vi "RCV Test_Hold and Measure Over Time_ksENA.vi"(0 "Semiconductor Module Context":T3, 1 "Hold Time(s)":dbl=1.0, 2 "Test Information":T6={"Exp Name"="Cold Switching", "Lot"="0233A", "Wafer"="15", "Die Type"="L22", "Die X "="6", "Die Y"="8", "Exp"="1", "Die X_Y"="8"}, 3 "# of Cycles":string, 5 "Sweep Settings":T4={"Start"=0.0, "Stop"=1.0, "Step"=0.0}, 7 "Test_Pins":T5={"RF_Pins"=["RF1", "RF2"], "Contact_Meas_Pins"=["RF1"], "Contact_Source_Pins"=["RF1"], "Sweep_Bias_Pins"=[]}, 9 "Averaging Count":i32=3, 11 "error in (no error)":errorcluster, 12 "Meas Type":T1, 13 "base path":path=path "C:/Users/Eddie.Rickey/Desktop/Test Data/Plots", 14 "Hold Down Current level":dbl=0.001 format="%#_13p") -> (4 "Time":dbl[](array[numeric]), 6 "ks5080A_Meaurements":T7, 15 "error out":errorcluster)   [LabVIEW 2013]
doc: "Initiates and fetches niVNA S11 measurements and converts it to a capacitance measurement."
uses:
  <vilib>/NI_TestStand_SemiconductorModule/NI_TestStand_Semiconductor_Module.lvlibp/PinMap/General/SemiconductorModuleContext.ctl
  Controls/Sweep Settings.ctl
  Controls/Test_Pins.ctl
  Controls/Test Information.ctl
  Controls/Meas Type.ctl
  Controls/ks5080A_Measurements.ctl
  <vilib>/NI_TestStand_SemiconductorModule/NI_TestStand_Semiconductor_Module.lvlibp
panel:
  in  "Tab Control":enum32{"Graphs", "Inputs", "Outputs"}(tab)
  out "Resistance over time":cluster{dbl[], dbl[]}(graph)
  out "Port Capacitance over time":cluster{dbl[], "P2_Capacitance":dbl[]}[](graph)
  out "Graph Cluster":T2
  out "Die Type":string
  out "Measurement":string
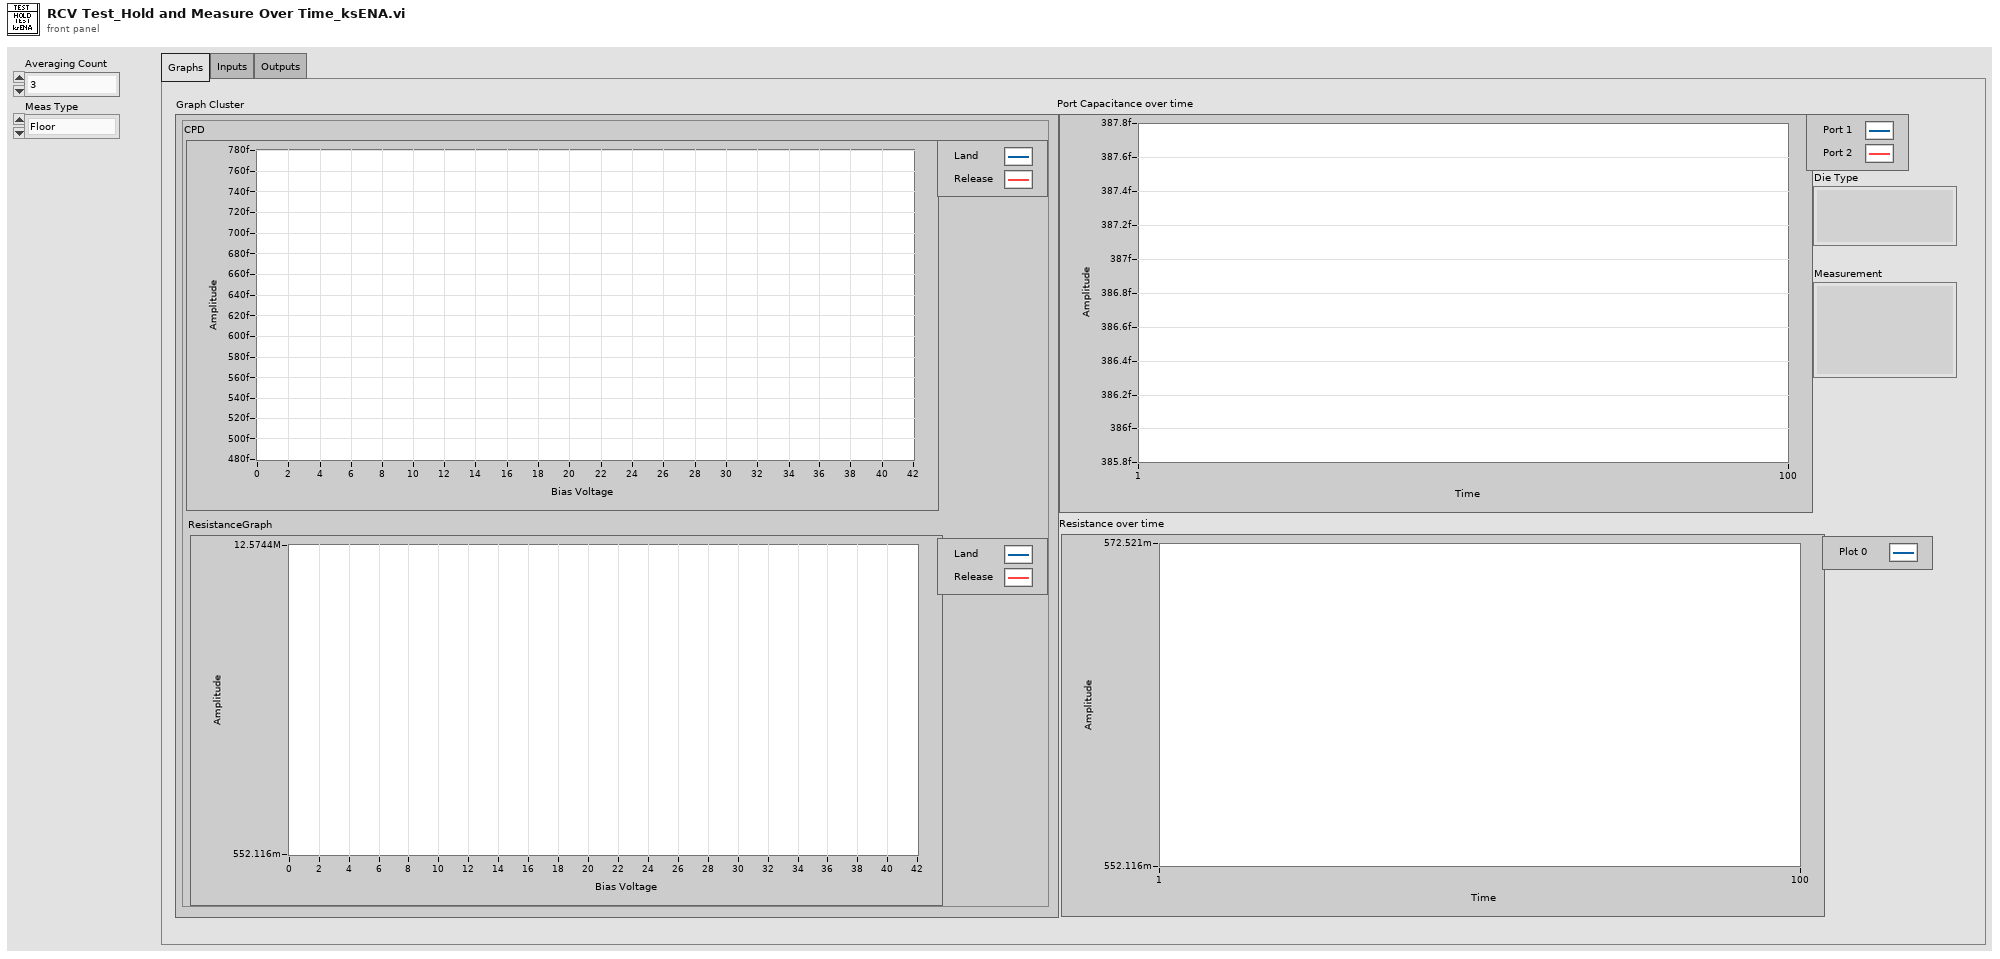
[diagram p1: front panel]
types:
  T1 = typedef "Meas Type.ctl" = enum16{"Floor", "Roof", "Buckling", "Charge Transfer"}
  T2 = cluster{"ResistanceGraph":cluster{dbl[], dbl[]}[], "CPD":cluster{dbl[], dbl[]}[]}
  T3 = typedef "NI_TestStand_Semiconductor_Module.lvlibp/SemiconductorModuleContext.ctl" = refnum<k7>
  T4 = typedef "Sweep Settings.ctl" = cluster{"Start":dbl, "Stop":dbl, "Step":dbl}
  T5 = typedef "Test_Pins.ctl" = cluster{"RF_Pins":string[], "Contact_Meas_Pins":string[], "Contact_Source_Pins":string[], "Sweep_Bias_Pins":string[]}
  T6 = typedef "Test Information.ctl" = cluster{"Exp Name":string, "Lot":string, "Wafer":string, "Die Type":string, "Die X ":string, "Die Y":string, "Exp":string, "Die X_Y":string}
  T7 = typedef "ks5080A_Measurements.ctl" = cluster{"Bias_Sweep_Setting":dbl[], "Bias_voltage measurements":dbl[], "Bias_current measurements":dbl[], "P1_Capacitance":dbl[], "P2_Capacitance":dbl[], "DMM_Measurement_V":dbl[], "Contact_Source Current measurements":dbl[], "Contact_Sink Current measurements":dbl[], "Calculated_Resistance":dbl[], "P3_Capacitance":dbl[], "Port 1_S_parm":string[], "Port 2_S_parm":string[], "Port 3_S_parm":string[]}
  T8 = enum16{"Initialize", "Insert Data into Array", "Get Data"}
  T9 = typedef "ENA_Marker Measurements.ctl" = cluster{"Port 1 Capacitance":dbl[], "Port 2 Capacitance":dbl[], "Port 3 Capacitance":dbl[], "Port 1_S_parm":string[], "Port 2_S_parm":string[], "Port 3_S_parm":string[]}
  T10 = typedef "imagedata.ctl" = cluster{"image type":i32, "image depth":i32, "image":u8[], "mask":u8[], "colors":u32[], "Rectangle":cluster{"left":i16, "top":i16, "right":i16, "bottom":i16}}
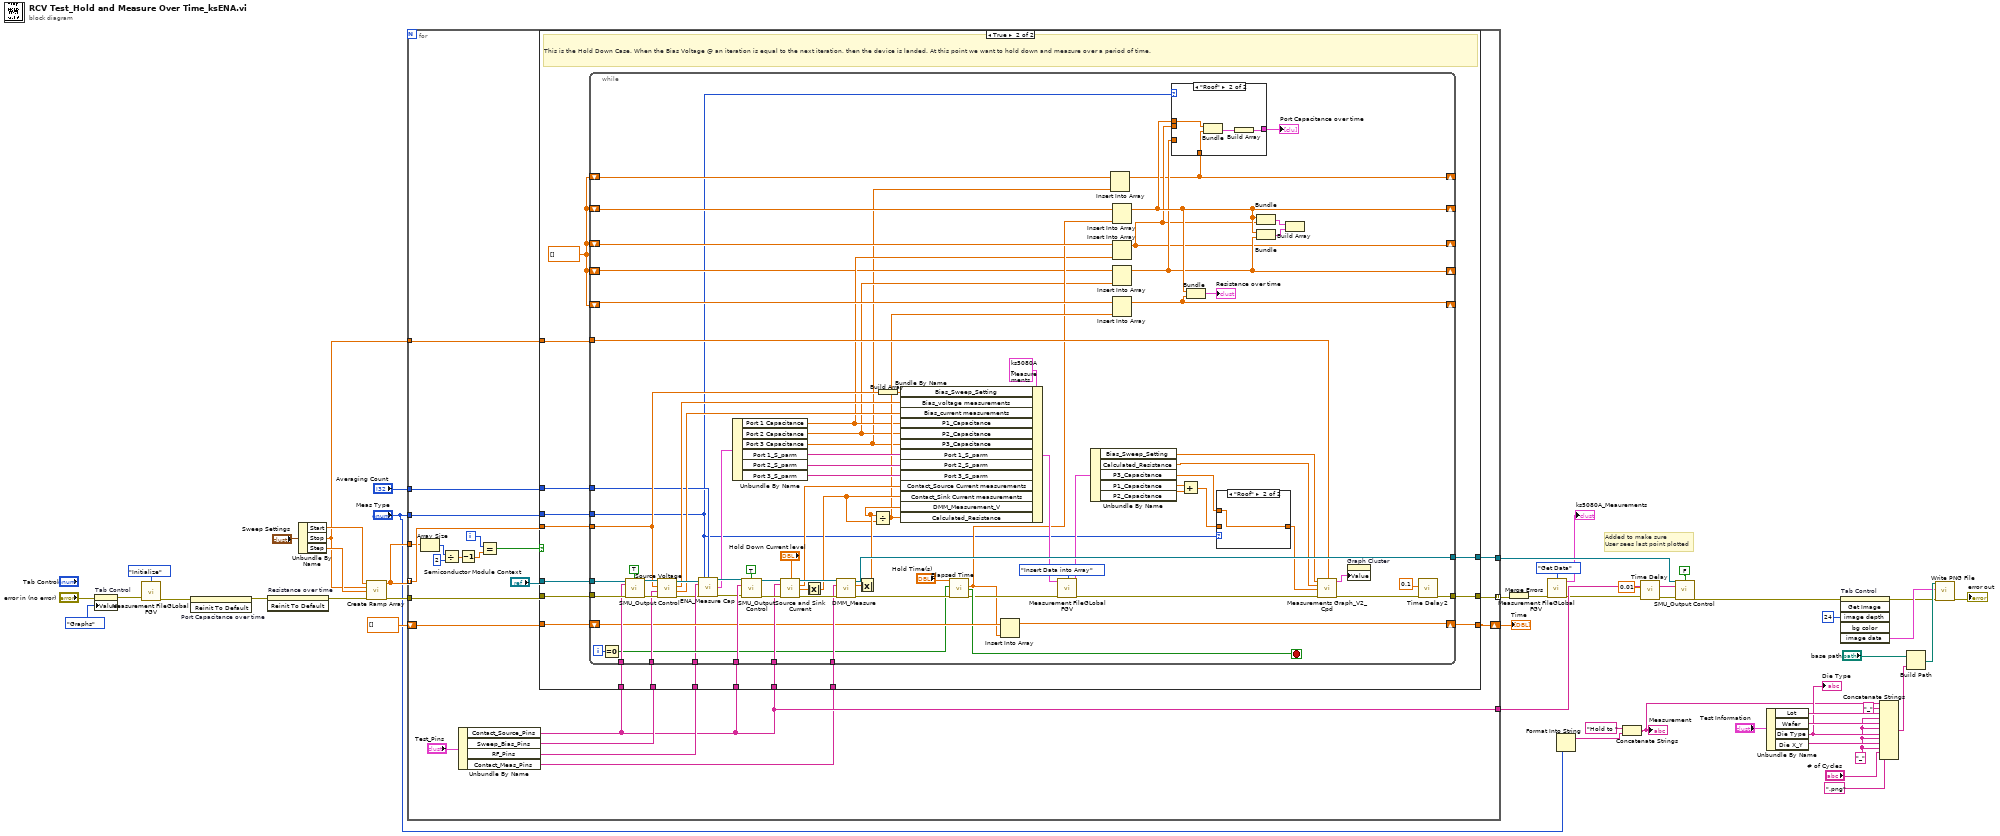
[diagram p0: block diagram]
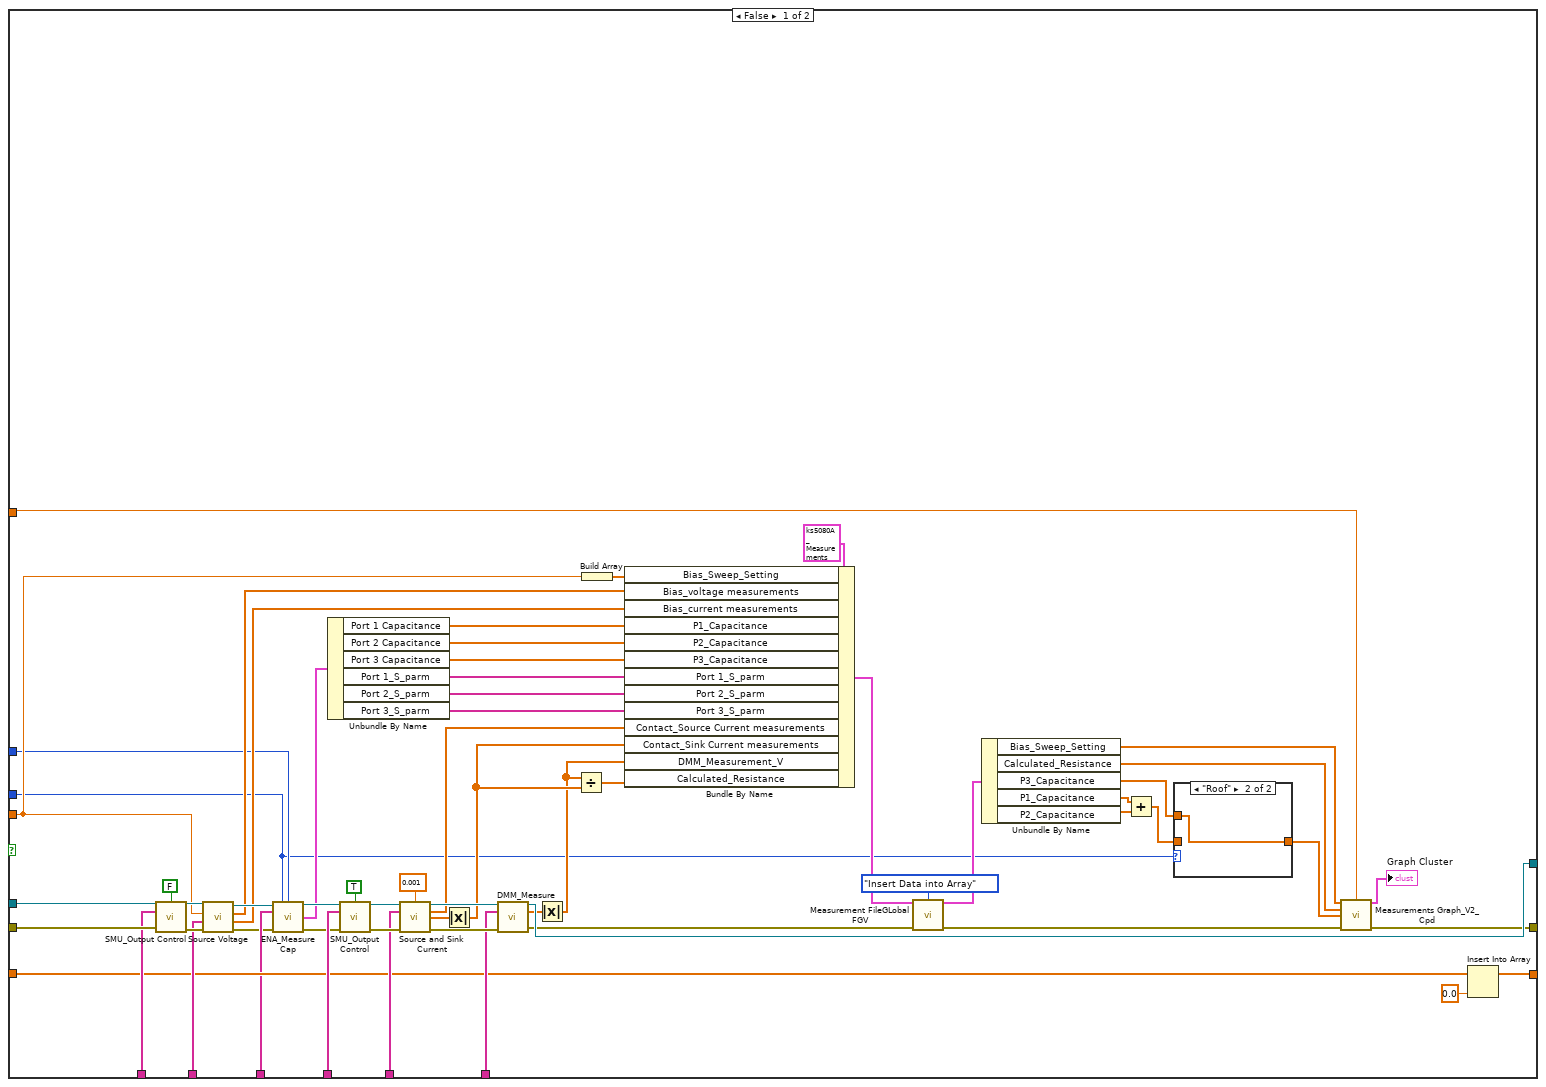
[diagram p2: hidden frame]
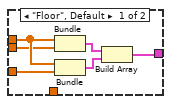
[diagram p4: hidden frame]
diagram:
  w3 = "_"
  # "Added to make sure \nUser sees last point plotted"
  n1 = property on="Tab Control" class="TabCtl (strict)"(error in="error in (no error)", "Value"=enum32{"Graphs", "Inputs", "Outputs"}."Graphs" ("Tab Control")) -> (error out=w14:errorcluster)  [unwired: 1 in, 1 out]
  n2 = call "Measurement FileGLobal FGV.vi"("Enum"=T8."Initialize", "Error In"=w14) -> ("Error Out"=w24:errorcluster)  [unwired: 12 in, 1 out]
  n3 = invoke on="Port Capacitance over time" class="XYGraph (strict)" method="Reinit To Default"(error in=w24) -> (error out=w26:errorcluster)  [unwired: 2 in, 2 out]
  n4 = invoke on="Resistance over time" class="XYGraph (strict)" method="Reinit To Default"(error in=w26) -> (error out=w25:errorcluster)  [unwired: 2 in, 2 out]
  n5 = Unbundle By Name("Sweep Settings") -> ("Start"=w45:dbl, "Stop"=w31:dbl, "Step"=w44:dbl)
  n6 = call "Create Ramp Array.vi"("Start"=w45, "Stop"=w31, "Step"=w44, "Error In"=w25) -> ("Ramp Pattern"=w27:dbl[], "Error Out"=w47:errorcluster)  [unwired: 10 in]
  n7 = for {
    tunnel: w27 -> [w58] mode=indexing
    tunnel: [w67] -> w20 mode=indexing
    tunnel: w47 -> [w68]
    tunnel: w31 -> [w57]
    tunnel: [w63] -> w30
    tunnel: [w61] -> w29
    shift-right: [w60] -> w28
    shift-left: dbl[] [] -> [w59]
    tunnel: w27 -> [w56]
    tunnel: "Averaging Count" -> [w49]
    tunnel: "Meas Type" -> [w48]
    i -> [w51]
    n8 = Array Size(array=w56) -> (size(s)=w55:i32)
    n9 = Divide(x=w55, y=2) -> (x/y=w53:dbl)
    n10 = Unbundle By Name("Test_Pins") -> ("Contact_Source_Pins"=w63:string[], "Sweep_Bias_Pins"=w65:string[], "RF_Pins"=w64:string[], "Contact_Meas_Pins"=w62:string[])
    n11 = Decrement(x=w53) -> (x-1=w52:dbl)
    n12 = Equal?(x=w51, y=w52) -> (x = y?=w50:bool)
    n13 = case shown="True" w50 {
      tunnel: [w82 w147] -> w67
      tunnel: w68 -> [w120 w148]
      tunnel: w58 -> [w100 w146]
      tunnel: w57 -> [w81 w145]
      tunnel: "Semiconductor Module Context" -> [w119 w144]
      tunnel: w63 -> [w117 w143]
      tunnel: w65 -> [w116 w142]
      tunnel: w64 -> [w107 w141]
      tunnel: w63 -> [w115 w140]
      tunnel: w63 -> [w114 w139]
      tunnel: w62 -> [w113 w138]
      tunnel: [w118 w137] -> w61
      tunnel: [w112 w136] -> w60
      tunnel: w59 -> [w111 w135]
      tunnel: w49 -> [w72 w134]
      tunnel: w48 -> [w71 w133]
      frame False {
        n14 = call "SMU_Output Control.vi"("Semiconductor Module Context"=w119, "output enabled?"=FALSE, "Pins"=w117, "error in (no error)"=w120) -> ("Semiconductor Module Context Out"=w128:T3, "error out"=w129:errorcluster)  [unwired: 10 in]
        n15 = call "Source Voltage.vi"("error in (no error)"=w129, "Pins"=w116, "voltage level"=w100, "Semiconductor Module Context"=w128) -> ("error out"=w106:errorcluster, "current measurements"=w97:dbl[], "voltage measurements"=w98:dbl[], "Semiconductor Module Context Out"=w103:T3)  [unwired: 4 in]
        n16 = call "ENA_Measure Cap.vi"("Semiconductor Module Context"=w103, "Meas Type"=w71, "Averaging Count"=w72, "Pins"=w107, "error in (no error)"=w106) -> ("Semiconductor Module Context Out"=w104:T3, "Marker Measurements"=w102:T9, "error out"=w105:errorcluster)  [unwired: 8 in]
        n17 = Unbundle By Name(w102) -> ("Port 1 Capacitance"=w95:dbl[], "Port 2 Capacitance"=w94:dbl[], "Port 3 Capacitance"=w93:dbl[], "Port 1_S_parm"=w92:string[], "Port 2_S_parm"=w91:string[], "Port 3_S_parm"=w90:string[])
        n18 = call "SMU_Output Control.vi"("Semiconductor Module Context"=w104, "output enabled?"=TRUE, "Pins"=w115, "error in (no error)"=w105) -> ("Semiconductor Module Context Out"=w121:T3, "error out"=w122:errorcluster)  [unwired: 10 in]
        n19 = call "Source and Sink Current.vi"("Semiconductor Module Context"=w121, "Current level"=0.001, "Pins"=w114, "error in (no error)"=w122) -> ("Semiconductor Module Context Out"=w123:T3, "Source Current measurements"=w89:dbl[], "Sink Current measurements"=w109:dbl[], "error out"=w124:errorcluster)  [unwired: 8 in]
        n20 = Absolute Value(x=w109) -> (abs(x)=w88:dbl[])
        n21 = call "DMM_Measure.vi"("Semiconductor Module Context"=w123, "Pins"=w113, "Error In"=w124) -> ("Semiconductor Module Context Out"=w118:T3, "Measurement"=w108:dbl[], "Error Out"=w86:errorcluster)  [unwired: 10 in]
        n22 = Absolute Value(x=w108) -> (abs(x)=w84:dbl[])
        n23 = Divide(x=w84, y=w88) -> (x/y=w87:dbl[])
        n24 = Build Array(w100) -> (w99:dbl[])
        n25 = Bundle By Name(cluster=T7 {"Bias_Sweep_Setting"=[], "Bias_voltage measurements"=[], "Bias_current measurements"=[], "P1_Capacitance"=[], "P2_Capacitance"=[], "DMM_Measurement_V"=[], "Contact_Source Current measurements"=[], "Contact_Sink Current measurements"=[], "Calculated_Resistance"=[], "P3_Capacitance"=[], "Port 1_S_parm"=[], "Port 2_S_parm"=[], "Port 3_S_parm"=[]} ("ks5080A_Meaurements"), "Bias_Sweep_Setting"=w99, "Bias_voltage measurements"=w98, "Bias_current measurements"=w97, "P1_Capacitance"=w95, "P2_Capacitance"=w94, "P3_Capacitance"=w93, "Port 1_S_parm"=w92, "Port 2_S_parm"=w91, "Port 3_S_parm"=w90, "Contact_Source Current measurements"=w89, "Contact_Sink Current measurements"=w88, "DMM_Measurement_V"=w84, "Calculated_Resistance"=w87) -> (w96:T7)
        n26 = call "Measurement FileGLobal FGV.vi"("New Measurements"=w96, "Enum"=T8."Insert Data into Array", "Error In"=w86) -> ("Combined Measurements"=w85:T7, "Error Out"=w83:errorcluster)  [unwired: 11 in]
        n27 = Unbundle By Name(w85) -> ("Bias_Sweep_Setting"=w79:dbl[], "Calculated_Resistance"=w78:dbl[], "P3_Capacitance"=w73:dbl[], "P1_Capacitance"=w77:dbl[], "P2_Capacitance"=w76:dbl[])
        n28 = Add(x=w77, y=w76) -> (x+y=w75:dbl[])
        n29 = case shown="\"Roof\"" w71 {
          tunnel: w75 -> [w130 _]
          tunnel: [w130 w131] -> w74
          tunnel: w73 -> [_ w131]
          frame "Floor", Default {
          }
          frame "Roof" {
          }
        }
        n30 = call "Measurements Graph_V2_Cpd.vi"("Bias Voltage"=w79, "Stop_V"=w81, "Resitance"=w78, "Cpd"=w74, "Error In"=w83) -> ("Graph Cluster"=→"Graph Cluster":T2, "Error Out"=w82:errorcluster)  [unwired: 9 in]
        n31 = Insert Into Array(array=w111, new element=0.0 ("new element/subarray")) -> (w112:dbl[])  [unwired: 1 in]
      }
      frame True {
        w132 = dbl[] []
        # "This is the Hold Down Case. When the Bias Voltage @ an iteration is equal to the next iteration, then the device is landed. At this point we want to hold down and measure over a period of time."
        n32 = while {
          tunnel: [w210] -> w147
          tunnel: w148 -> [w219]
          tunnel: w146 -> [w190]
          tunnel: w145 -> [w174]
          tunnel: w144 -> [w218]
          tunnel: w143 -> [w217]
          tunnel: w142 -> [w216]
          tunnel: w141 -> [w197]
          tunnel: w140 -> [w215]
          tunnel: w139 -> [w214]
          tunnel: w138 -> [w213]
          tunnel: [w212] -> w137
          shift-right: [w200] -> w136
          shift-left: w135 -> [w209]
          shift-right: [w161] -> _
          shift-left: w132 -> [w202]
          shift-right: [w155] -> _
          shift-left: w132 -> [w201]
          shift-right: [w157] -> _
          shift-left: w132 -> [w165]
          tunnel: w134 -> [w159]
          tunnel: w133 -> [w151]
          shift-right: [w156] -> _
          shift-left: w132 -> [w163]
          shift-right: [w152] -> _
          shift-left: w132 -> [w154]
          i -> [w206]
          stop <- w208 stop-if-true
          n33 = Equal To 0?(x=w206) -> (x = 0?=w205:bool)
          n34 = call "SMU_Output Control.vi"("Semiconductor Module Context"=w218, "output enabled?"=TRUE, "Pins"=w217, "error in (no error)"=w219) -> ("Semiconductor Module Context Out"=w228:T3, "error out"=w229:errorcluster)  [unwired: 10 in]
          n35 = call "Source Voltage.vi"("error in (no error)"=w229, "Pins"=w216, "voltage level"=w190, "Semiconductor Module Context"=w228) -> ("error out"=w149:errorcluster, "current measurements"=w192:dbl[], "voltage measurements"=w193:dbl[], "Semiconductor Module Context Out"=w195:T3)  [unwired: 4 in]
          n36 = call "ENA_Measure Cap.vi"("Semiconductor Module Context"=w195, "Meas Type"=w151, "Averaging Count"=w159, "Pins"=w197, "error in (no error)"=w149) -> ("Semiconductor Module Context Out"=w194:T3, "Marker Measurements"=w189:T9, "error out"=w196:errorcluster)  [unwired: 8 in]
          n37 = Unbundle By Name(w189) -> ("Port 1 Capacitance"=w164:dbl[], "Port 2 Capacitance"=w162:dbl[], "Port 3 Capacitance"=w153:dbl[], "Port 1_S_parm"=w188:string[], "Port 2_S_parm"=w187:string[], "Port 3_S_parm"=w186:string[])
          n38 = call "SMU_Output Control.vi"("Semiconductor Module Context"=w194, "output enabled?"=TRUE, "Pins"=w215, "error in (no error)"=w196) -> ("Semiconductor Module Context Out"=w221:T3, "error out"=w222:errorcluster)  [unwired: 10 in]
          n39 = call "Source and Sink Current.vi"("Semiconductor Module Context"=w221, "Current level"="Hold Down Current level", "Pins"=w214, "error in (no error)"=w222) -> ("Semiconductor Module Context Out"=w223:T3, "Source Current measurements"=w185:dbl[], "Sink Current measurements"=w204:dbl[], "error out"=w224:errorcluster)  [unwired: 8 in]
          n40 = Absolute Value(x=w204) -> (abs(x)=w183:dbl[])
          n41 = call "DMM_Measure.vi"("Semiconductor Module Context"=w223, "Pins"=w213, "Error In"=w224) -> ("Semiconductor Module Context Out"=w212:T3, "Measurement"=w203:dbl[], "Error Out"=w220:errorcluster)  [unwired: 10 in]
          n42 = Absolute Value(x=w203) -> (abs(x)=w184:dbl[])
          n43 = Divide(x=w184, y=w183) -> (x/y=w169:dbl[])
          n44 = Build Array(w190) -> (w191:dbl[])
          n45 = Bundle By Name(cluster=T7 {"Bias_Sweep_Setting"=[], "Bias_voltage measurements"=[], "Bias_current measurements"=[], "P1_Capacitance"=[], "P2_Capacitance"=[], "DMM_Measurement_V"=[], "Contact_Source Current measurements"=[], "Contact_Sink Current measurements"=[], "Calculated_Resistance"=[], "P3_Capacitance"=[], "Port 1_S_parm"=[], "Port 2_S_parm"=[], "Port 3_S_parm"=[]} ("ks5080A_Meaurements"), "Bias_Sweep_Setting"=w191, "Bias_voltage measurements"=w193, "Bias_current measurements"=w192, "P1_Capacitance"=w164, "P2_Capacitance"=w162, "P3_Capacitance"=w153, "Port 1_S_parm"=w188, "Port 2_S_parm"=w187, "Port 3_S_parm"=w186, "Contact_Source Current measurements"=w185, "Contact_Sink Current measurements"=w183, "DMM_Measurement_V"=w184, "Calculated_Resistance"=w169) -> (w182:T7)
          n46 = call "Elapsed Time"("Time Target (s)"="Hold Time(s)", "Reset"=w205, "error in (no error)"=w220) -> ("Elapsed Time (s)"=w167:dbl, "Time has Elapsed"=w208:bool, "error out"=w199:errorcluster)  [unwired: 9 in, 5 out]
          n47 = Insert Into Array(array=w209, new element=w167) -> (w200:dbl[])  [unwired: 1 in]
          n48 = call "Measurement FileGLobal FGV.vi"("New Measurements"=w182, "Enum"=T8."Insert Data into Array", "Error In"=w199) -> ("Combined Measurements"=w173:T7, "Error Out"=w177:errorcluster)  [unwired: 11 in]
          n49 = Unbundle By Name(w173) -> ("Bias_Sweep_Setting"=w172:dbl[], "Calculated_Resistance"=w171:dbl[], "P3_Capacitance"=w178:dbl[], "P1_Capacitance"=w181:dbl[], "P2_Capacitance"=w180:dbl[])
          n50 = Insert Into Array(array=w154, new element=w153) -> (w152:dbl[])  [unwired: 1 in]
          n51 = Insert Into Array(array=w165, new element=w167) -> (w157:dbl[])  [unwired: 1 in]
          n52 = Insert Into Array(array=w201, new element=w164) -> (w155:dbl[])  [unwired: 1 in]
          n53 = Insert Into Array(array=w163, new element=w162) -> (w156:dbl[])  [unwired: 1 in]
          n54 = Insert Into Array(array=w202, new element=w169) -> (w161:dbl[])  [unwired: 1 in]
          n55 = case shown="\"Roof\"" w151 {
            tunnel: [w233 w238] -> w158
            tunnel: w157 -> [w232 w237]
            tunnel: w155 -> [w231 _]
            tunnel: w156 -> [w230 _]
            tunnel: w152 -> [_ w236]
            frame "Floor", Default {
              n56 = Bundle(w232, w231) -> (w235:cluster{dbl[], dbl[]})  [unwired: 1 in]
              n57 = Bundle(w232, w230) -> (w234:cluster{dbl[], dbl[]})  [unwired: 1 in]
              n58 = Build Array(w235, w234) -> (w233:cluster{dbl[], dbl[]}[])
            }
            frame "Roof" {
              n59 = Bundle(w237, w236) -> (w239:cluster{dbl[], dbl[]})  [unwired: 1 in]
              n60 = Build Array(w239) -> (w238:cluster{dbl[], dbl[]}[])
            }
          }
          "Port Capacitance over time" <- w158
          n61 = Add(x=w181, y=w180) -> (x+y=w179:dbl[])
          n62 = Bundle(w157, w161) -> (→"Resistance over time":cluster{dbl[], dbl[]})  [unwired: 1 in]
          n63 = case shown="\"Roof\"" w151 {
            tunnel: w179 -> [w240 _]
            tunnel: [w240 w241] -> w170
            tunnel: w178 -> [_ w241]
            frame "Floor", Default {
            }
            frame "Roof" {
            }
          }
          n64 = Bundle(w157, w155) -> (w168:cluster{dbl[], dbl[]})  [unwired: 1 in]
          n65 = Bundle(w157, w156) -> (w166:cluster{dbl[], dbl[]})  [unwired: 1 in]
          n66 = Build Array(w168, w166) -> ()  [unwired: 1 out]
          n67 = call "Measurements Graph_V2_Cpd.vi"("Bias Voltage"=w172, "Stop_V"=w174, "Resitance"=w171, "Cpd"=w170, "Error In"=w177) -> ("Graph Cluster"=w175:T2, "Error Out"=w176:errorcluster)  [unwired: 9 in]
          n68 = property on="Graph Cluster" class="Clust (strict)"("Value"=w175) -> ()  [unwired: 2 in, 2 out]
          n69 = call "Time Delay2"("error in (no error)"=w176, "Delay Time (s)"=0.1) -> ("error out"=w210:errorcluster)  [unwired: 9 in]
        }
      }
    }
  }
  "Time" <- w28
  n70 = Merge Errors(w20) -> (w19:errorcluster)
  n71 = call "Measurement FileGLobal FGV.vi"("Enum"=T8."Get Data", "Error In"=w19) -> ("Combined Measurements"=→"ks5080A_Meaurements":T7, "Error Out"=w18:errorcluster)  [unwired: 12 in]
  n72 = Format Into String("Meas Type") -> (resulting string=w7:string)  [unwired: 3 in, 1 out]
  n73 = Concatenate Strings("Hold to " ("string"), w7) -> (w5:string)
  "Measurement" <- w5
  n74 = call "Time Delay"("error in (no error)"=w18, "Delay Time (s)"=0.01) -> ("error out"=w41:errorcluster)  [unwired: 9 in]
  n75 = call "SMU_Output Control.vi"("Semiconductor Module Context"=w29, "output enabled?"=FALSE, "Pins"=w30, "error in (no error)"=w41) -> ("error out"=w10:errorcluster)  [unwired: 10 in, 1 out]
  n76 = Unbundle By Name("Test Information") -> ("Lot"=w39:string, "Wafer"=w38:string, "Die Type"=w37:string, "Die X_Y"=w36:string)
  "Die Type" <- w37
  n77 = invoke on="Tab Control" class="TabCtl (strict)" method="Get Image"(error in=w10, "image depth"=24 ("Image Depth")) -> (error out=w9:errorcluster, "image data"=w11:T10)  [unwired: 4 in, 4 out]
  n78 = Concatenate Strings(w5, "_" ("string"), w39, w3, w38, w3, w37, w3, w36, w3, "# of Cycles", ".png" ("string")) -> (w35:string)
  n79 = Build Path(base path="base path", name or relative path=w35) -> (appended path=w33:path)
  n80 = call <vilib>:"Write PNG File.vi"("error in (no error)"=w9, "image data"=w11, "path to PNG file"=w33) -> ("error out"=→"error out":errorcluster)  [unwired: 7 in, 1 out]
